vi "wait for data.vi"(8 "error in":errorcluster, 9 "timeout in ms (-1)":i32=-1, 11 "refnum in":T1) -> (0 "error out":errorcluster, 1 "data out":variant, 2 "command":string, 3 "refnum out":T1)   [LabVIEW 2020, in "Publisher Subscriber.lvlib"]
uses:
  Publisher Subscriber.lvlib
  Controls/node refnum.ctl
  Controls/node dvr data.ctl
  Controls/data cluster.ctl
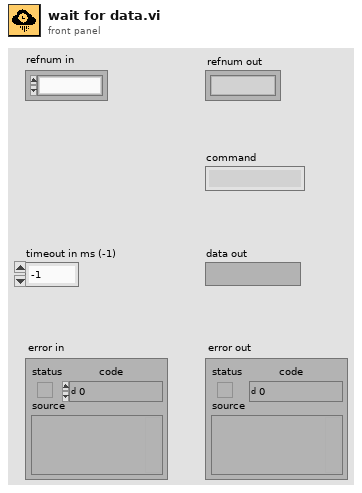
[diagram p1: front panel]
types:
  T1 = typedef "Publisher Subscriber.lvlib/node refnum.ctl" = refnum<k1>
  T2 = typedef "Publisher Subscriber.lvlib/node dvr data.ctl" = cluster{"queue ref":refnum<queue>, "subscription map ref":refnum<data-value>, "Command":string, "Data":variant, "Subscriptions []":set{string}, "variable dvr refs":refnum<data-value>}
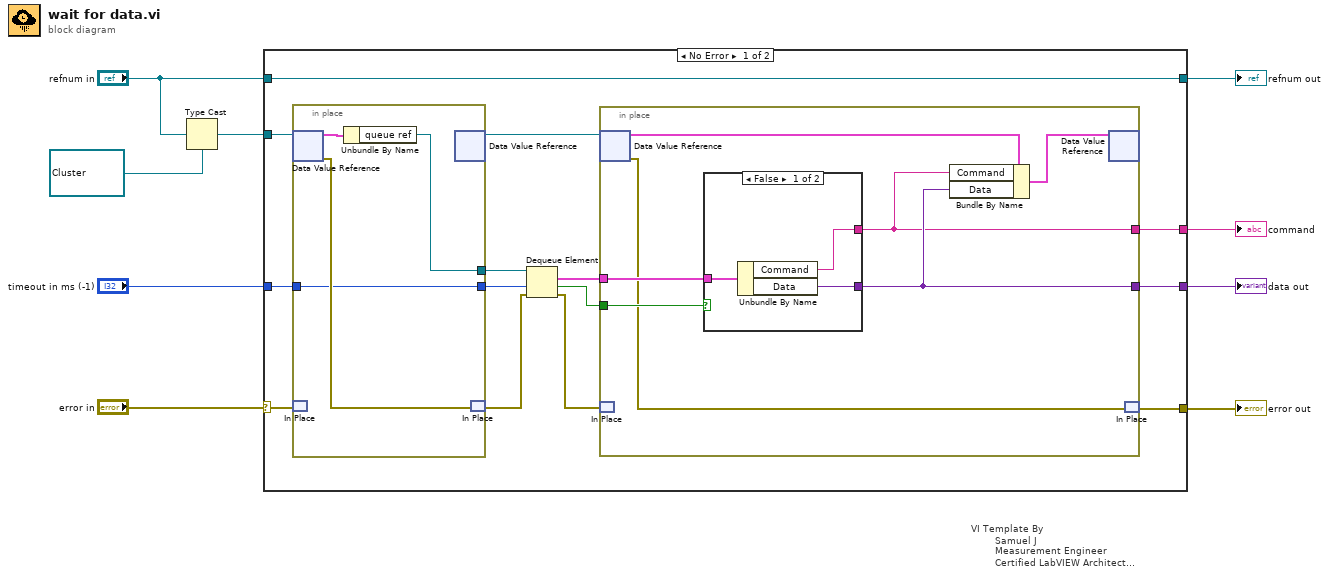
[diagram p0: block diagram]
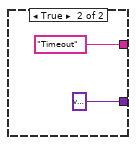
[diagram p2: hidden frame]
diagram:
  n1 = Type Cast(type=refnum<data-value> refnum ("data value reference"), x="refnum in") -> (*(type *) &x=w6:refnum<data-value>)
  n2 = case "VI Template By\n        Samuel J\n        Measurement Engineer\n        Certified LabVIEW Architect\n        Vestas Technology R&D Chennai" shown="No Error" "error in" {
    selector: "error in" -> [w16 w41]
    tunnel: [w20 w41] -> w8
    tunnel: w6 -> [w18 _]
    tunnel: [w23 w40] -> w5
    tunnel: "refnum in" -> [w23 w40]
    tunnel: "timeout in ms (-1)" -> [w19 _]
    tunnel: [w22 _] -> w2
    tunnel: [w21 _] -> w1
    frame No Error {
      n3 = in-place {
        in-place-border: w19 -> [w24]
        in-place-border: [w25] -> w15
        in-place-border: [w24] -> w14
        n4 = in-place-dvr #1(w18) -> (w27:T2, w26:errorcluster)
        n5 = in-place-match #2(w16) -> ()  [unwired: 1 out]
        n6 = Unbundle By Name(w27) -> ("queue ref"=w25:refnum<queue>)
        n7 = in-place-dvr #1() -> (w17:refnum<data-value>)  [unwired: 1 in, 1 out]
        n8 = in-place-match #2(w26) -> (w11:errorcluster)
      }
      n9 = Dequeue Element(queue=w15, timeout in ms (-1)=w14, error in (no error)=w11) -> (element=w13:cluster{"Command":string, "Data":variant}, timed out?=w12:bool, error out=w10:errorcluster)  [unwired: 1 out]
      n10 = in-place {
        in-place-border: [w32] -> w21
        in-place-border: [w31] -> w22
        in-place-border: w13 -> [w30]
        in-place-border: w12 -> [w29]
        n11 = in-place-dvr #3(w17) -> (w33:T2, w28:errorcluster)
        n12 = in-place-match #4(w10) -> ()  [unwired: 1 out]
        n13 = case shown="False" w29 {
          tunnel: w30 -> [w37 _]
          tunnel: [w36 "Timeout" ("Command")] -> w31
          tunnel: [w35 variant ("Data")] -> w32
          frame False {
            n14 = Unbundle By Name(w37) -> ("Command"=w36:string, "Data"=w35:variant)
          }
          frame True {
          }
        }
        n15 = Bundle By Name(cluster=w33, "Command"=w31, "Data"=w32) -> (w34:T2)
        n16 = in-place-dvr #3(w34) -> ()  [unwired: 2 out]
        n17 = in-place-match #4(w28) -> (w20:errorcluster)
      }
    }
    frame Error {
    }
  }
  "error out" <- w8
  "refnum out" <- w5
  "data out" <- w1
  "command" <- w2
